vi "Read Trace Message.vi"(8 "error in (no error)":errorcluster, 11 "Trace in":refnum<class "Trace.lvclass">) -> (0 "error out":errorcluster, 2 "Trace Message":string, 3 "Trace out":refnum<class "Trace.lvclass">)   [LabVIEW 2014, in "Robot Actor Framework.lvlib" / "Trace.lvlib" / "Trace.lvclass"]
uses:
  Trace.lvclass
  Trace.lvclass/Trace.ctl
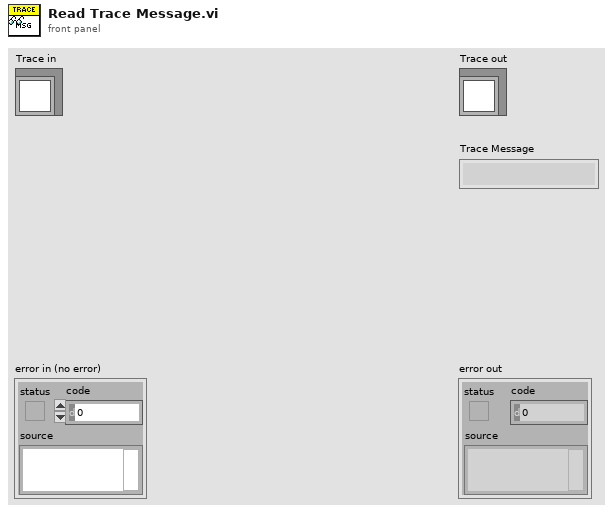
[diagram p1: front panel]
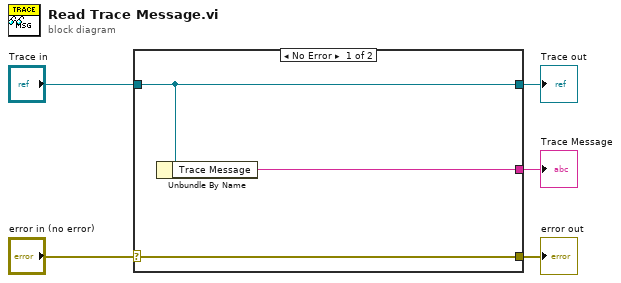
[diagram p0: block diagram]
diagram:
  n1 = case shown="No Error" "error in (no error)" {
    selector: "error in (no error)" -> [w8 w9]
    tunnel: [w8 w9] -> w4
    tunnel: [w7 w10] -> w2
    tunnel: "Trace in" -> [w7 w10]
    tunnel: [w6 _] -> w1
    frame No Error {
      n2 = Unbundle By Name(w7) -> ("Trace Message"=w6:string)
    }
    frame Error {
    }
  }
  "error out" <- w4
  "Trace out" <- w2
  "Trace Message" <- w1
